vi "Add Bold Tags.vi"(9 "Selection in":T1, 11 "Value in":string) -> (1 "Selection out":T1, 3 "Value out":string)   [LabVIEW 2023, in "VI Properties Editor.lvlib"]
doc: "Adds HTML bold tags to <B> Value in</B> around <B>Selection in</B>, and modifies the selection to select the same substring as before the addition of the tags."
uses:
  <vilib>/Utility/miscctls.llb/LVSelectionTypeDef.ctl
  VI Properties Editor.lvlib
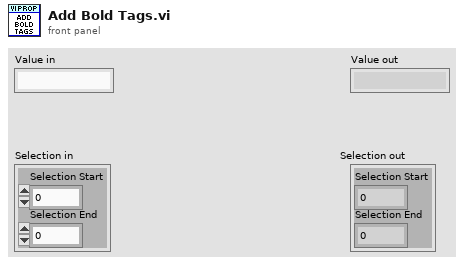
[diagram p1: front panel]
types:
  T1 = typedef "LVSelectionTypeDef.ctl" = cluster{"Selection Start":u32, "Selection End":u32}
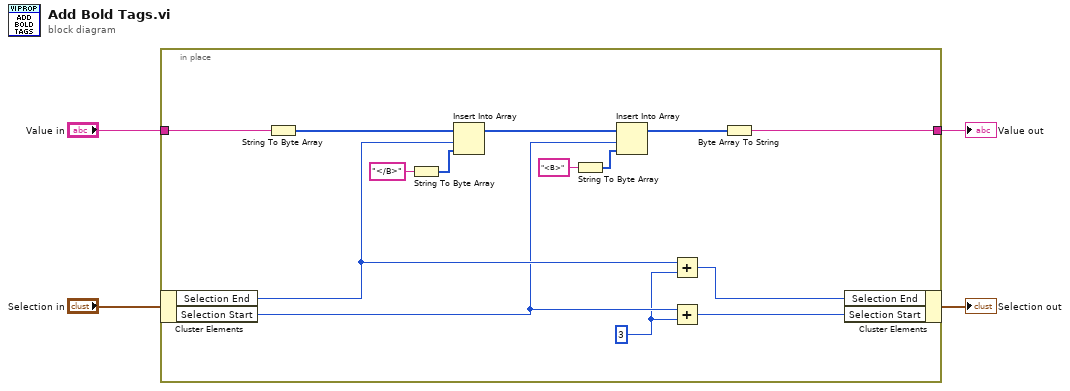
[diagram p0: block diagram]
diagram:
  n1 = in-place {
    in-place-border: "Value in" -> [w18]
    in-place-border: [w10] -> w1
    w7 = u32 3 ("y")
    n2 = in-place-cluster #1("Selection in") -> ("Selection End"=w9:u32, "Selection Start"=w8:u32)
    n3 = String To Byte Array(string=w18) -> (unsigned byte array=w15:u8[])
    n4 = String To Byte Array(string="</B>") -> (unsigned byte array=w13:u8[])
    n5 = Insert Into Array(array=w15, index=w9, new element=w13) -> (w14:u8[])
    n6 = String To Byte Array(string="<B>") -> (unsigned byte array=w12:u8[])
    n7 = Insert Into Array(array=w14, index=w8, new element=w12) -> (w11:u8[])
    n8 = Add(x=w9, y=w7) -> (x+y=w6:u32)
    n9 = Add(x=w8, y=w7) -> (x+y=w5:u32)
    n10 = Byte Array To String(unsigned byte array=w11) -> (string=w10:string)
    n11 = in-place-cluster #1("Selection End"=w6, "Selection Start"=w5) -> (→"Selection out":T1)
  }
  "Value out" <- w1
